vi "Parse iCalendar.vi"(8 "error in":errorcluster, 11 "iCalendar string":string) -> (0 "error out":errorcluster, 1 "Last Data":T1, 5 "Events out":T1[](array[typedef]))   [LabVIEW 2020]
doc: "Read iCalendar File VI opens an iCalendar file and extracts the most important information out of it."
uses:
  Extract iCalendar String.ctl
panel:
  out "result string":string
  out "Tokens array":string[](array[string])
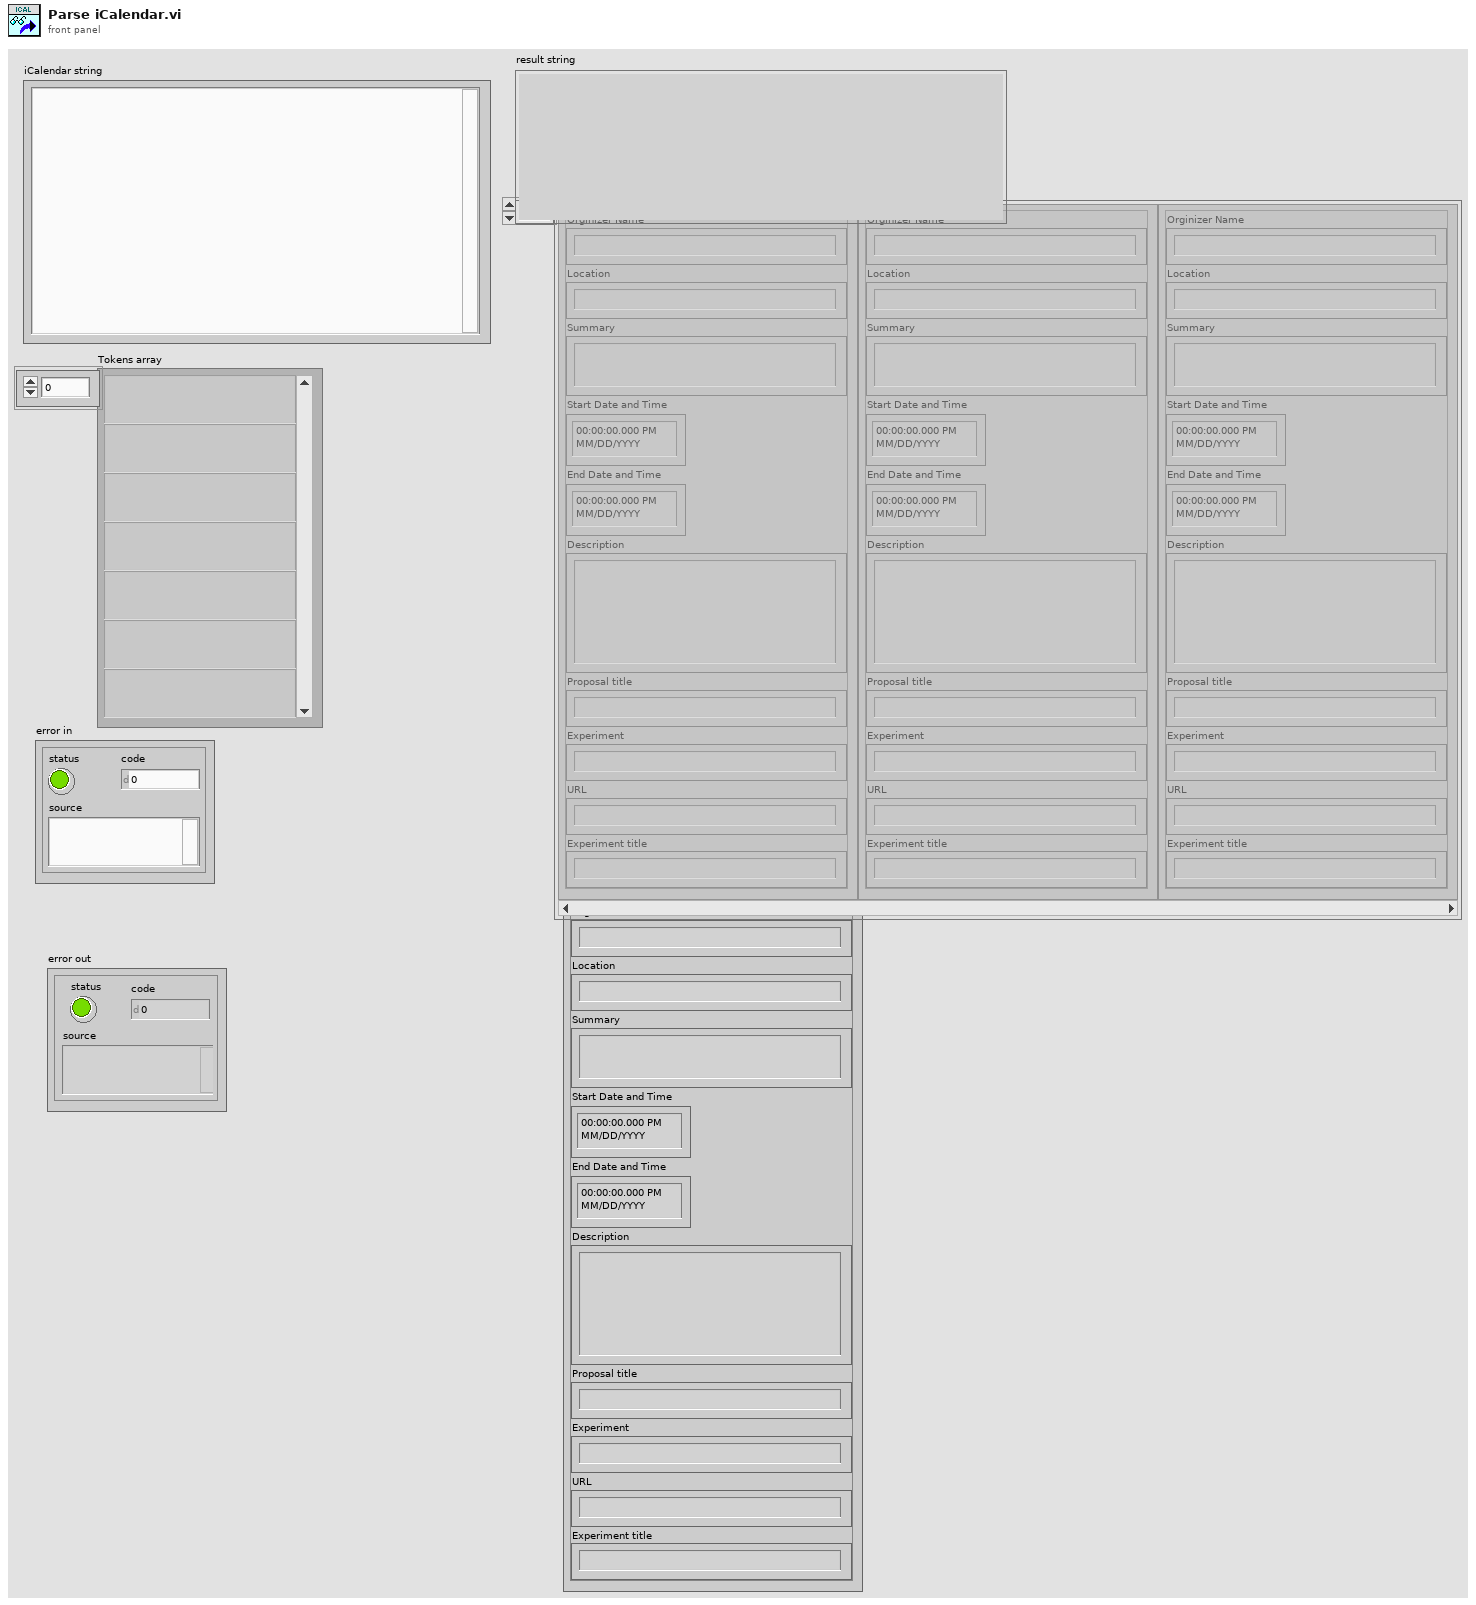
[diagram p1: front panel]
types:
  T1 = typedef "Extract iCalendar String.ctl" = cluster{"Orginizer Name":string, "Location":string, "Summary":string, "Start Date and Time":timestamp, "End Date and Time":timestamp, "Description":string, "Proposal title":string, "Experiment":string, "URL":string, "Experiment title":string}
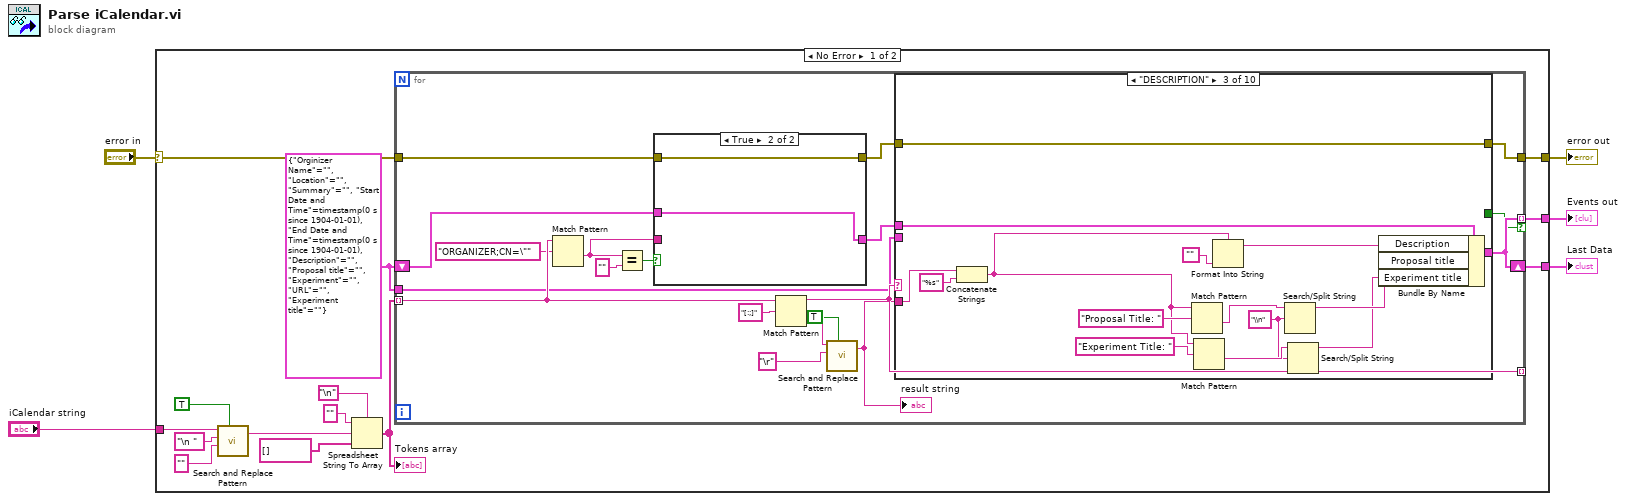
[diagram p0: block diagram]
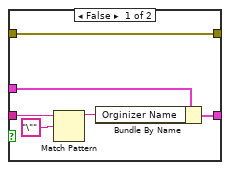
[diagram p2: hidden frame]
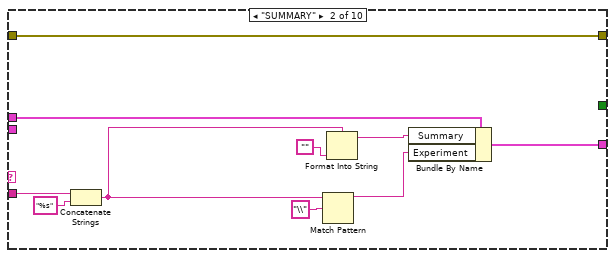
[diagram p4: hidden frame]
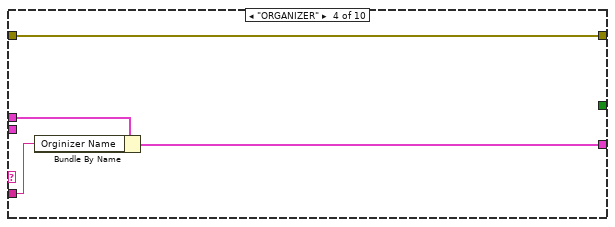
[diagram p5: hidden frame]
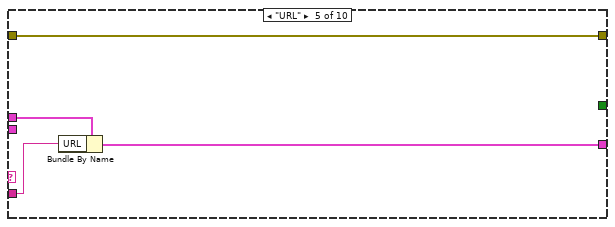
[diagram p6: hidden frame]
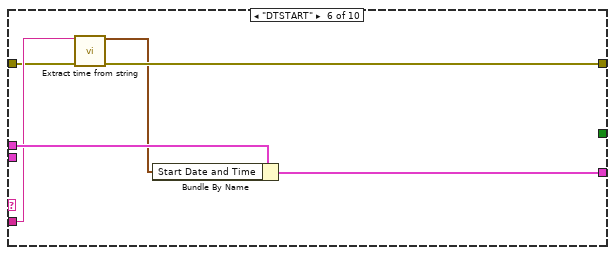
[diagram p7: hidden frame]
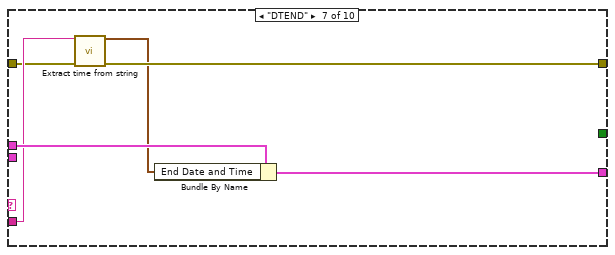
[diagram p8: hidden frame]
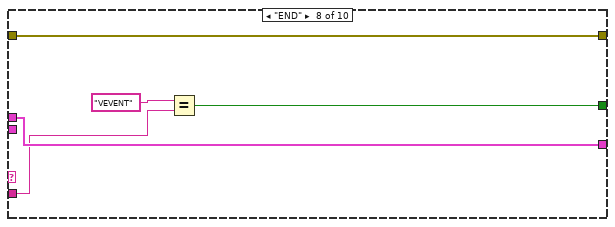
[diagram p9: hidden frame]
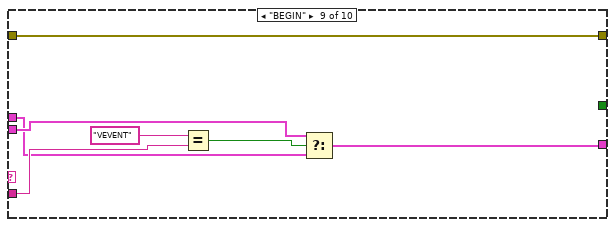
[diagram p10: hidden frame]
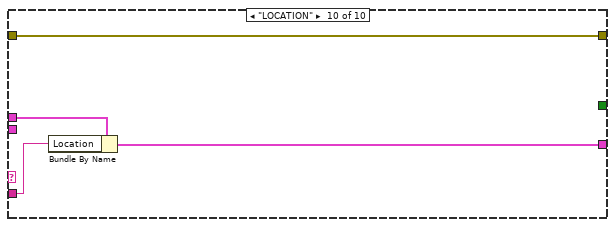
[diagram p11: hidden frame]
diagram:
  n1 = case shown="No Error" "error in" {
    selector: "error in" -> [w13 w110]
    tunnel: [w15 w110] -> w4
    tunnel: [w14 _] -> w3
    tunnel: [w12 _] -> w2
    tunnel: "iCalendar string" -> [w6 _]
    frame No Error {
      w7 = T1 {"Orginizer Name"="", "Location"="", "Summary"="", "Start Date and Time"=timestamp(0 s since 1904-01-01), "End Date and Time"=timestamp(0 s since 1904-01-01), "Description"="", "Proposal title"="", "Experiment"="", "URL"="", "Experiment title"=""} ("output cluster")
      n2 = call <vilib>:"Search and Replace Pattern.vi"("string"=w6, "regular expression (\"\")"="\n " ("regular expression (\"\")"), "replace string (\"\")"="" ("replace string (\"\")"), "replace all? (F)"=TRUE) -> ("result string"=w9:string)  [unwired: 1 in, 1 out]
      n3 = Spreadsheet String To Array(delimiter (Tab)="\n", format string="", spreadsheet string=w9, array type (2D Dbl)=string[] []) -> (array=w16:string[])
      "Tokens array" <- w16
      n4 = for {
        tunnel: w16 -> [w37] mode=indexing
        tunnel: [w38] -> _ mode=indexing
        shift-right: [w26] -> w14
        shift-left: w7 -> [w32]
        tunnel: w13 -> [w29]
        tunnel: [w27] -> w15
        tunnel: [w26] -> w12 mode=indexing if=w25
        tunnel: w7 -> [w24]
        n5 = Match Pattern(string=w37, regular expression="ORGANIZER;CN=\"") -> (after substring=w31:string)  [unwired: 1 in, 3 out]
        n6 = Equal?(x=w31, y="" ("format string")) -> (x = y?=w34:bool)
        n7 = case shown="True" w34 {
          tunnel: w32 -> [w44 w46]
          tunnel: w31 -> [w42 _]
          tunnel: [w43 w46] -> w30
          tunnel: w29 -> [w39 w45]
          tunnel: [w39 w45] -> w28
          frame False {
            n8 = Match Pattern(string=w42, regular expression="\"") -> (before substring=w41:string)  [unwired: 1 in, 3 out]
            n9 = Bundle By Name(cluster=w44, "Orginizer Name"=w41) -> (w43:T1)
          }
          frame True {
          }
        }
        n10 = Match Pattern(string=w37, regular expression="[:;]" ("format string")) -> (before substring=w38:string, after substring=w22:string)  [unwired: 1 in, 2 out]
        n11 = call <vilib>:"Search and Replace Pattern.vi"("string"=w22, "regular expression (\"\")"="\r" ("regular expression (\"\")"), "replace all? (F)"=TRUE) -> ("result string"=w21:string)  [unwired: 2 in, 1 out]
        "result string" <- w21
        n12 = case shown="\"DESCRIPTION\"" w38 {
          tunnel: w21 -> [_ w53 w69 w76 w80 w85 w91 w97 w105 w107]
          tunnel: w30 -> [w48 w58 w73 w77 w81 w87 w93 w98 w100 w109]
          tunnel: [w48 w57 w72 w75 w79 w86 w92 w98 w99 w108] -> w26
          tunnel: w28 -> [w47 w56 w71 w74 w78 w84 w90 w94 w103 w106]
          tunnel: [w47 w56 w71 w74 w78 w83 w89 w94 w103 w106] -> w27
          tunnel: [_ _ _ _ _ _ _ w95 _ _] -> w25
          tunnel: w24 -> [_ _ _ _ _ _ _ _ w101 _]
          frame Default {
          }
          frame "SUMMARY" {
            n13 = Concatenate Strings(w53, "%s" ("string")) -> (w51:string)
            n14 = Match Pattern(string=w51, regular expression="\\") -> (before substring=w49:string)  [unwired: 1 in, 3 out]
            n15 = Format Into String(format string=w51, "") -> (resulting string=w52:string)  [unwired: 2 in, 1 out]
            n16 = Bundle By Name(cluster=w58, "Summary"=w52, "Experiment"=w49) -> (w57:T1)
          }
          frame "DESCRIPTION" {
            w60 = "\\n" ("regular expression")
            n17 = Concatenate Strings(w69, "%s" ("string")) -> (w62:string)
            n18 = Match Pattern(string=w62, regular expression="Proposal Title: ") -> (after substring=w64:string)  [unwired: 1 in, 3 out]
            n19 = Match Pattern(string=w62, regular expression="Experiment Title: ") -> (after substring=w61:string)  [unwired: 1 in, 3 out]
            n20 = Format Into String(format string=w62, "") -> (resulting string=w70:string)  [unwired: 2 in, 1 out]
            n21 = Search/Split String(string=w64, search string/char (-)=w60) -> (substring before match=w65:string)  [unwired: 1 in, 2 out]
            n22 = Search/Split String(string=w61, search string/char (-)=w60) -> (substring before match=w59:string)  [unwired: 1 in, 2 out]
            n23 = Bundle By Name(cluster=w73, "Description"=w70, "Proposal title"=w65, "Experiment title"=w59) -> (w72:T1)
          }
          frame "ORGANIZER" {
            n24 = Bundle By Name(cluster=w77, "Orginizer Name"=w76) -> (w75:T1)
          }
          frame "URL" {
            n25 = Bundle By Name(cluster=w81, "URL"=w80) -> (w79:T1)
          }
          frame "DTSTART" {
            n26 = call "Extract time from string.vi"("ics time string"=w85, "Error In"=w84) -> ("Time and Date"=w82:timestamp, "Error Out"=w83:errorcluster)  [unwired: 12 in]
            n27 = Bundle By Name(cluster=w87, "Start Date and Time"=w82) -> (w86:T1)
          }
          frame "DTEND" {
            n28 = call "Extract time from string.vi"("ics time string"=w91, "Error In"=w90) -> ("Time and Date"=w88:timestamp, "Error Out"=w89:errorcluster)  [unwired: 12 in]
            n29 = Bundle By Name(cluster=w93, "End Date and Time"=w88) -> (w92:T1)
          }
          frame "END" {
            n30 = Equal?(x="VEVENT", y=w97) -> (x = y?=w95:bool)
          }
          frame "BEGIN" {
            n31 = Equal?(x="VEVENT", y=w105) -> (x = y?=w102:bool)
            n32 = Select(t=w101, s=w102, f=w100) -> (s? t:f=w99:T1)
          }
          frame "LOCATION" {
            n33 = Bundle By Name(cluster=w109, "Location"=w107) -> (w108:T1)
          }
        }
      }
    }
    frame Error {
    }
  }
  "error out" <- w4
  "Last Data" <- w3
  "Events out" <- w2
